vi "Translator.Control.Fglb.vi"(7 "Action":T3, 8 "error in (no error)":errorcluster, 10 "Controls in":T1[](array[typedef]), 11 "VI name":string) -> (0 "error out":errorcluster, 2 "Controls out":T1[](array[typedef]))   [LabVIEW 2016]
uses:
  Translator.ControlData.ctl
  Translator.ControlTypes.ctl
  Translator.Control.Fglb.Action.vi
  Translator.Global.vi
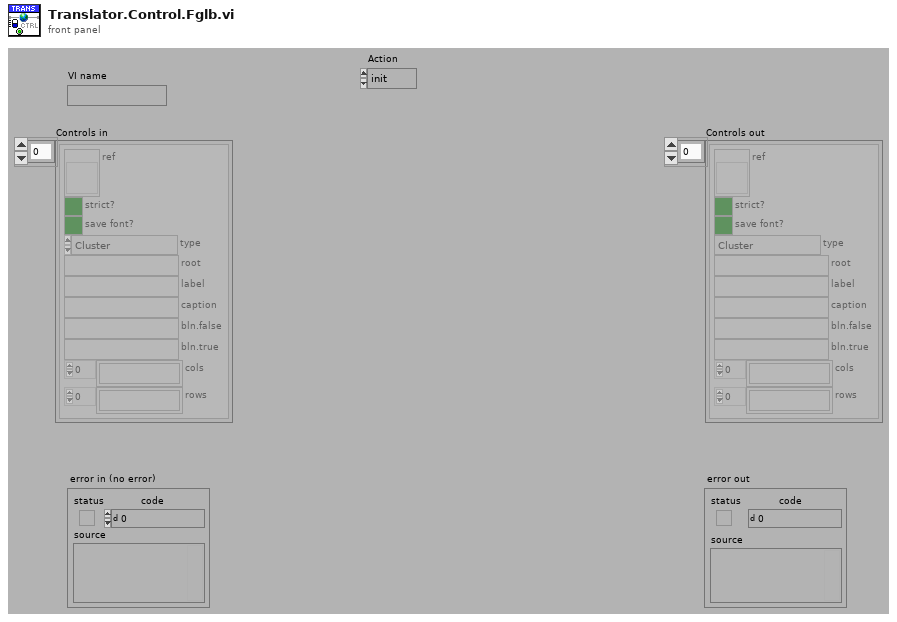
[diagram p1: front panel]
types:
  T1 = typedef "Translator.ControlData.ctl" = cluster{"ref":refnum<vi>, "strict?":bool, "save font?":bool, "type":T2, "root":string, "label":string, "caption":string, "bln.false":string, "bln.true":string, "cols":string[], "rows":string[]}
  T2 = typedef "Translator.ControlTypes.ctl" = enum16{"Cluster", "Array", "Boolean", "Ring", "String", "Tab", "Listbox", "Multicolumn listbox", "Table", "Tree", "Other"}
  T3 = typedef "Translator.Control.Fglb.Action.vi" = enum16{"init", "set", "get", "clear"}
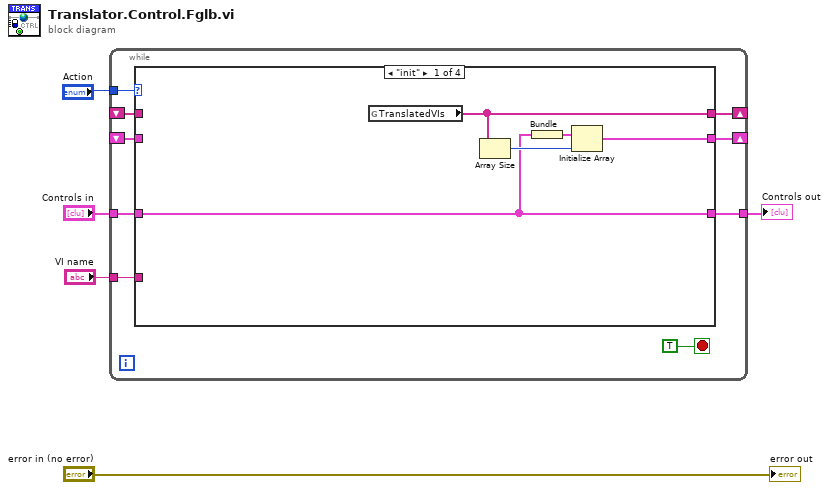
[diagram p0: block diagram]
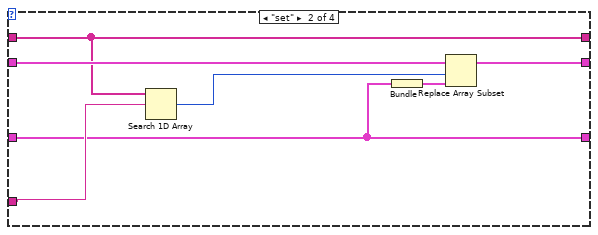
[diagram p2: hidden frame]
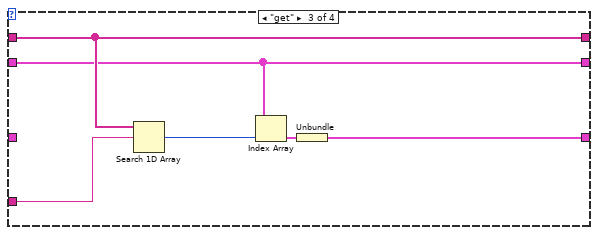
[diagram p3: hidden frame]
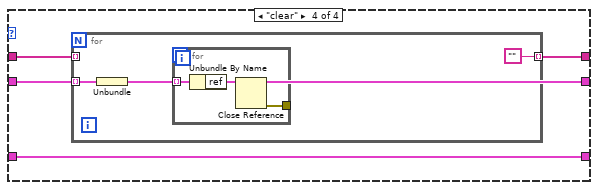
[diagram p4: hidden frame]
diagram:
  n1 = while {
    tunnel: "Action" -> [w13]
    tunnel: "Controls in" -> [w12]
    tunnel: [w11] -> w2
    tunnel: "VI name" -> [w10]
    shift-right: [w9] -> _
    shift-left: _ -> [w8]
    shift-right: [w6] -> _
    shift-left: _ -> [w7]
    stop <- TRUE stop-if-true
    n2 = case shown="\"init\"" w13 {
      tunnel: [w17 w20 w28 w33] -> w11
      tunnel: w12 -> [w17 w20 _ w33]
      tunnel: w10 -> [_ w24 w32 _]
      tunnel: [w19 w23 w31 w35] -> w9
      tunnel: w8 -> [_ w23 w31 w36]
      tunnel: w7 -> [_ w26 w30 w34]
      tunnel: [w15 w25 w30 w34] -> w6
      frame "init" {
        n3 = global read "Translator.Global.vi" "TranslatedVIs"() -> (w19:string[])
        n4 = Array Size(array=w19) -> (size(s)=w18:i32)
        n5 = Bundle("Controls in"=w17) -> (w16:cluster{"Controls in":T1[]})  [unwired: 1 in]
        n6 = Initialize Array(w16, w18) -> (w15:cluster{"Controls in":T1[]}[])
      }
      frame "set" {
        n7 = Search 1D Array(1D array=w23, element=w24) -> (index of element=w22:i32)  [unwired: 1 in]
        n8 = Bundle("Controls in"=w20) -> (w21:cluster{"Controls in":T1[]})  [unwired: 1 in]
        n9 = Replace Array Subset(array=w26, new element=w21, index=w22) -> (w25:cluster{"Controls in":T1[]}[])
      }
      frame "get" {
        n10 = Search 1D Array(1D array=w31, element=w32) -> (index of element=w27:i32)  [unwired: 1 in]
        n11 = Index Array(array=w30, index=w27) -> (element=w29:cluster{"Controls in":T1[]})
        n12 = Unbundle(w29) -> ("Controls in"=w28:T1[])
      }
      frame "clear" {
        n13 = for {
          tunnel: w34 -> [w39] mode=indexing
          tunnel: w36 -> [_] mode=indexing
          tunnel: [""] -> w35 mode=indexing
          n14 = Unbundle(w39) -> ("Controls in"=w38:T1[])
          n15 = for {
            tunnel: w38 -> [w42] mode=indexing
            tunnel: [w40] -> _
            n16 = Unbundle By Name(w42) -> ("ref"=w41:refnum<vi>)
            n17 = Close Reference(reference=w41) -> (error out=w40:errorcluster)  [unwired: 1 in]
          }
        }
      }
    }
  }
  "Controls out" <- w2
  "error out" <- "error in (no error)"
